vi "Read 3D Scatter Property Array.vi"(8 "error in (no error)":errorcluster, 11 "3D Scatter.lvclass in":refnum<class "3D Scatter.lvclass">) -> (0 "error out":errorcluster, 2 "3D Scatter Property Array":T1, 3 "3D Scatter.lvclass out":refnum<class "3D Scatter.lvclass">)   [LabVIEW 2017, in "3D Scatter.lvclass"]
uses:
  <vilib>/Math Plots/3D Math Plots/3D Scatter/3D Scatter/3D Scatter.lvclass
  <vilib>/Math Plots/3D Math Plots/3D Scatter/3D Scatter/Typedef/3D Scatter Property Array.ctl
  <vilib>/Math Plots/3D Math Plots/3D Scatter/3D Scatter/Typedef/3D Scatter Property.ctl
  <vilib>/Math Plots/3D Math Plots/3D Plot/3D Plot/Typedef/Sprite Type.ctl
  <vilib>/Math Plots/3D Math Plots/3D Plot/3D Plot/Typedef/Color Ramp Cluster.ctl
  <vilib>/Math Plots/3D Math Plots/3D Scatter/3D Scatter/3D Scatter.lvclass/3D Scatter.ctl
  <vilib>/Math Plots/3D Math Plots/3D Plot/3D Plot/3D Plot.lvclass
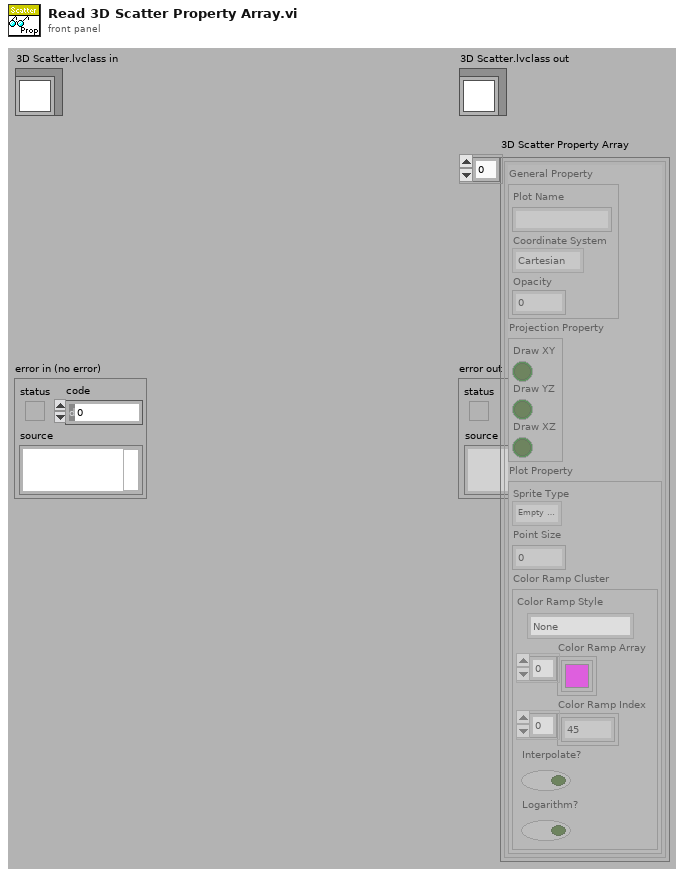
[diagram p1: front panel]
types:
  T1 = typedef "3D Scatter.lvclass/3D Scatter Property Array.ctl" = T2[]
  T2 = typedef "3D Scatter.lvclass/3D Scatter Property.ctl" = cluster{"General Property":cluster{"Plot Name":string, "Coordinate System":enum16{"Cartesian", "Cylindrical", "Spherical"}, "Opacity":sgl}, "Projection Property":cluster{"Draw XY":bool, "Draw YZ":bool, "Draw XZ":bool}, "Plot Property":cluster{"Sprite Type":T3, "Point Size":sgl, "Color Ramp Cluster":T4}}
  T3 = typedef "3D Plot.lvclass/Sprite Type.ctl" = enum16{"None", "Empty Square", "Solid Square", "Empty Diamond", "Solid Diamond", "Empty Circle", "Solid Circle", "Asterisk", "Bold X", "Wireframe Sphere", "Solid Sphere", "Wireframe Cube", "Solid Cube"}
  T4 = typedef "3D Plot.lvclass/Color Ramp Cluster.ctl" = cluster{"Color Ramp Style":enum16{"None", "Shaded", "Color spectrum", "Grey scale", "Custom"}, "Color Ramp Array":u32[], "Color Ramp Index":i32[], "Interpolate?":bool, "Logarithm?":bool}
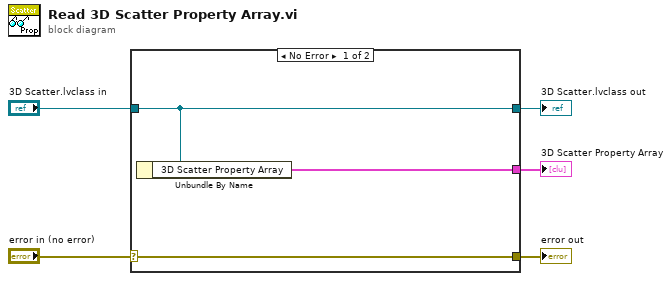
[diagram p0: block diagram]
diagram:
  n1 = case shown="No Error" "error in (no error)" {
    selector: "error in (no error)" -> [w8 w9]
    tunnel: [w8 w9] -> w4
    tunnel: [w7 w10] -> w2
    tunnel: "3D Scatter.lvclass in" -> [w7 w10]
    tunnel: [w6 _] -> w1
    frame No Error {
      n2 = Unbundle By Name(w7) -> ("3D Scatter Property Array"=w6:T1)
    }
    frame Error {
    }
  }
  "error out" <- w4
  "3D Scatter.lvclass out" <- w2
  "3D Scatter Property Array" <- w1
